vi "CRYCustom Unit Text.vi"(11 "Custom unit info":T1 {"dB ref" format="%.2f"}) -> (3 "Unit indicator text":string)   [LabVIEW 2013]
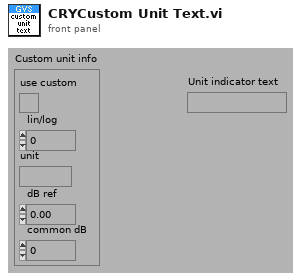
[diagram p1: front panel]
types:
  T1 = cluster{"use custom":bool, "lin/log":u16, "unit":string, "dB ref":dbl, "common dB":u16}
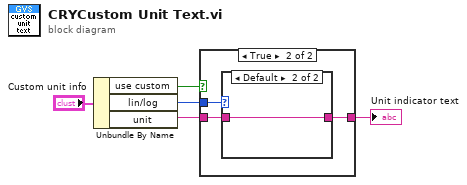
[diagram p0: block diagram]
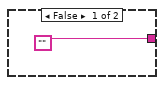
[diagram p2: hidden frame]
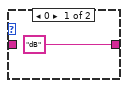
[diagram p3: hidden frame]
diagram:
  n1 = Unbundle By Name("Custom unit info") -> ("use custom"=w4:bool, "lin/log"=w3:u16, "unit"=w2:string)
  n2 = case shown="True" w4 {
    tunnel: w3 -> [_ w9]
    tunnel: w2 -> [_ w8]
    tunnel: ["" w7] -> w1
    frame False {
    }
    frame True {
      n3 = case shown="Default" w9 {
        tunnel: w8 -> [_ w11]
        tunnel: ["dB" w11] -> w7
        frame 0 {
        }
        frame Default {
        }
      }
    }
  }
  "Unit indicator text" <- w1
